vi "Fluence in Tile.vi"(0 "Analyze Fluence in":refnum<class "Analyze Fluence.lvclass">, 5 "Image in":T1, 7 "Energy":dbl, 9 "Create Overlay(T)?":bool, 11 "error in (no error)":errorcluster) -> (4 "Analyze Fluence out":refnum<class "Analyze Fluence.lvclass">, 6 "Image Dst Out":T1, 8 "Max Fluence J/cm^2":dbl, 10 "fluence infos":T2[](array[typedef]), 15 "error out":errorcluster)   [LabVIEW 2014, in "Analyze.lvlib" / "Analyze Fluence.lvclass"]
uses:
  Analyze Fluence.lvclass
  <vilib>/vision/NI_Vision_Development_Module.lvlib
  Fluence Info.ctl
  <vilib>/vision/Image Controls.llb/IMAQ Image.ctl
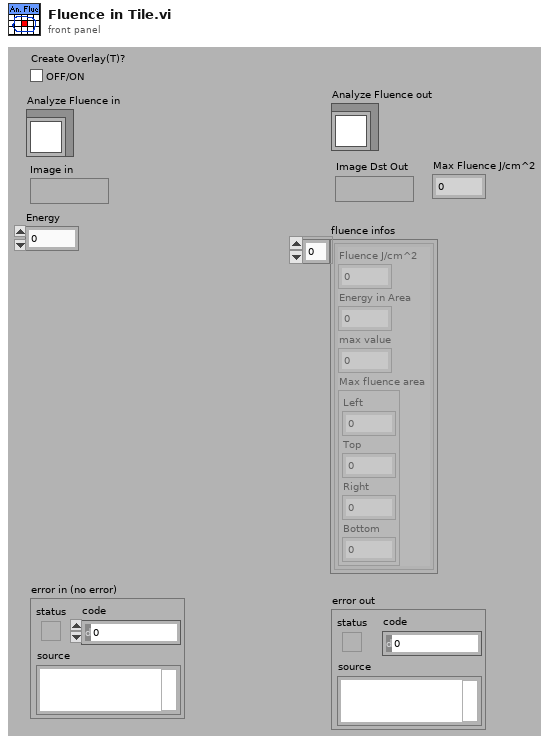
[diagram p1: front panel]
types:
  T1 = typedef "IMAQ Image.ctl" = refnum<image>
  T2 = typedef "Analyze.lvlib/Analyze Fluence.lvclass/Fluence Info.ctl" = cluster{"Fluence J/cm^2":dbl, "Energy in Area":dbl, "max value":i64, "Max fluence area":cluster{"Left":i32, "Top":i32, "Right":i32, "Bottom":i32}}
  T3 = cluster{"Left":i32, "Top":i32, "Right":i32, "Bottom":i32}
  T4 = typedef "Image Type" = u32
  T5 = typedef "ROI Descriptor" = cluster{"Global Rectangle":i32[], "Contours":cluster{"ID":enum32{"External", "Internal"}, "Type":u32, "Coordinates":i32[]}[]}
  T6 = cluster{"Desired Font (Application)":enum16{"User-specified Font", "Application Font", "System Font", "Dialog Font"}, "[User-specified Font]":cluster{"Font Name":string, "Size":i16, "Strikeout?":bool, "Italic?":bool, "Underline?":bool, "Outline?":bool, "Shadow?":bool, "Bold?":bool, "Rotation Angle":dbl}, "Horizontal Alignment":i16, "Vertical Alignment":i16}
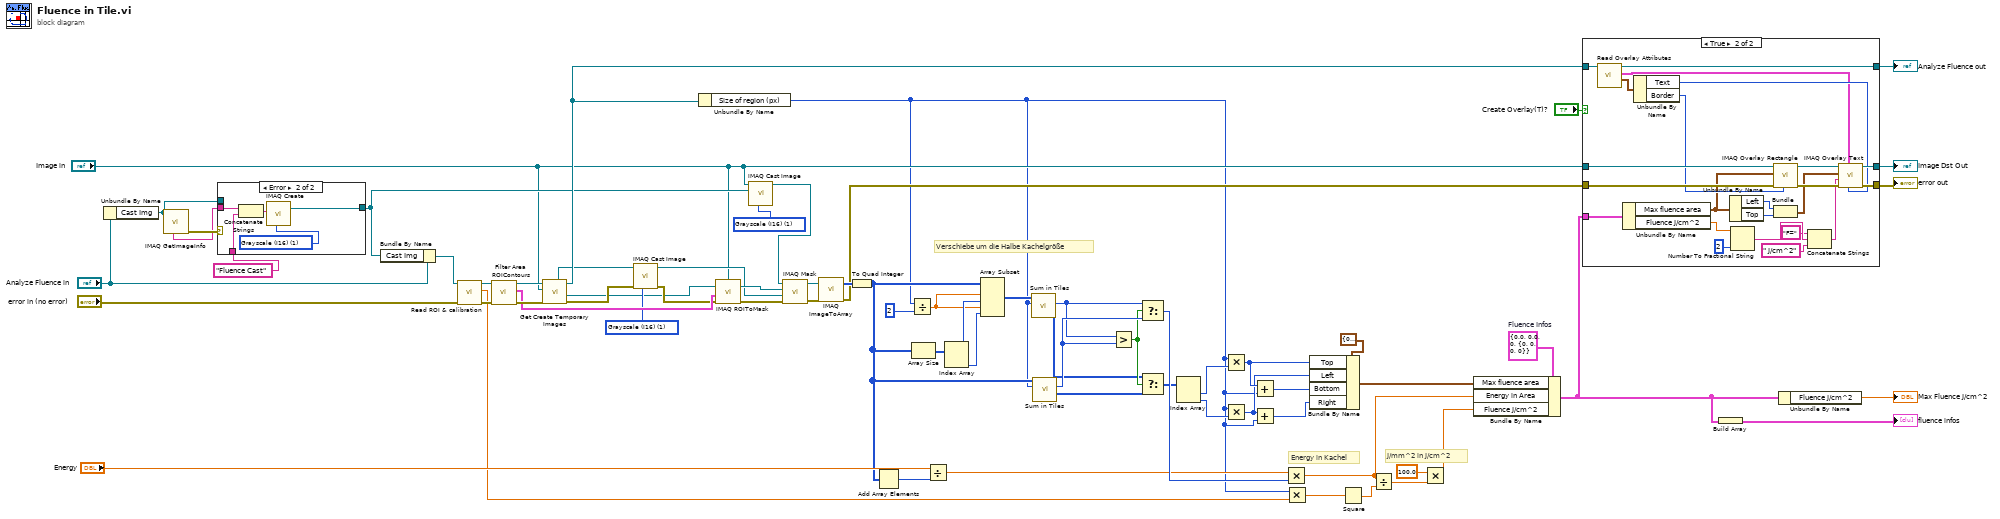
[diagram p0: block diagram]
diagram:
  w8 = T2 {"Fluence J/cm^2"=0.0, "Energy in Area"=0.0, "max value"=0, "Max fluence area"={"Left"=0, "Top"=0, "Right"=0, "Bottom"=0}}  # Fluence Infos
  w44 = T4 1 items=["Grayscale (U8)", "Grayscale (I16)", "Grayscale (SGL)", "Complex (CSG)", "RGB (U32)", "HSL (U32)", "RGB (U64)", "Grayscale (U16)"] ("Image Type")
  w54 = T4 1 items=["Grayscale (U8)", "Grayscale (I16)", "Grayscale (SGL)", "Complex (CSG)", "RGB (U32)", "HSL (U32)", "RGB (U64)", "Grayscale (U16)"] ("Image Type")
  # "Verschiebe um die Halbe Kachelgröße"
  # "J/mm^2 in J/cm^2"
  # "Energy in Kachel"
  n1 = Unbundle By Name("Analyze Fluence in") -> ("Cast Img"=w49:T1)
  n2 = call "IMAQ GetImageInfo"("Image"=w49) -> ("error out"=w52:errorcluster, "Image Name"=w51:string)  [unwired: 3 in, 6 out]
  n3 = case shown="Error" w52 {
    tunnel: w51 -> [_ w77]
    tunnel: "Fluence Cast" -> [_ w75]
    tunnel: [w73 w74] -> w47
    tunnel: w49 -> [w73 _]
    frame No Error {
    }
    frame Error {
      w78 = T4 1 items=["Grayscale (U8)", "Grayscale (I16)", "Grayscale (SGL)", "Complex (CSG)", "RGB (U32)", "HSL (U32)", "RGB (U64)", "Grayscale (U16)"] ("Image Type")
      n4 = Concatenate Strings(w77, w75) -> (w76:string)
      n5 = call "IMAQ Create"("Image Name"=w76, "Image Type"=w78) -> ("New Image"=w74:T1)  [unwired: 3 in, 1 out]
    }
  }
  n6 = Bundle By Name(cluster="Analyze Fluence in", "Cast Img"=w47) -> (w48:refnum<class "Analyze Fluence.lvclass">)
  n7 = call-dynamic "Read ROI & calibration.vi"("error in (no error)"="error in (no error)", "Analyze BaseClass in"=w48) -> ("error out"=w60:errorcluster, "calibration mm/px"=w32:dbl, "Analyze BaseClass out"=w63:refnum<class "Analyze Fluence.lvclass">)  [unwired: 6 in, 1 out]
  n8 = call-dynamic "Filter Area ROIContours.vi"("error in (no error)"=w60, "Analyze BaseClass in"=w63) -> ("error out"=w59:errorcluster, "ROI of Area type"=w56:T5, "Analyze BaseClass out"=w62:refnum<class "Analyze Fluence.lvclass">)  [unwired: 7 in]
  n9 = call-dynamic "Get Create Temporary Images.vi"("error in (no error)"=w59, "Image in"="Image in", "Analyze BaseClass in"=w62) -> ("error out"=w43:errorcluster, "image mask"=w28:T1, "Analyze BaseClass out"=w64:refnum<class "Analyze Fluence.lvclass">, "masked image"=w46:T1)  [unwired: 4 in, 1 out]
  n10 = call "IMAQ Cast Image"("Image Type"=w44, "error in (no error)"=w43, "Image Src"=w46) -> ("error out"=w42:errorcluster, "Image Dst Out"=w45:T1)  [unwired: 7 in]
  n11 = Unbundle By Name(w64) -> ("Size of region (px)"=w9:i32)
  n12 = call "IMAQ ROIToMask"("error in (no error)"=w42, "ROI Descriptor"=w56, "Image"=w28, "Image Model"="Image in") -> ("error out"=w67:errorcluster, "Image Out"=w71:T1)  [unwired: 2 in, 1 out]
  n13 = call "IMAQ Cast Image"("Image Type"=w54, "Image Dst"=w47, "Image Src"="Image in") -> ("Image Dst Out"=w55:T1)  [unwired: 7 in, 1 out]
  n14 = call "IMAQ Mask"("error in (no error)"=w67, "Image Dst"=w45, "Image Mask"=w71, "Image Src"=w55) -> ("error out"=w23:errorcluster, "Image Dst Out"=w24:T1)  [unwired: 1 in]
  n15 = call "IMAQ ImageToArray"("error in (no error)"=w23, "Image"=w24) -> ("error out"=w22:errorcluster, "Image Pixels (I16)"=w58:i16[][])  [unwired: 2 in, 3 out]
  n16 = To Quad Integer(1:w58) -> (0:w57:i64[][])
  n17 = Add Array Elements(numeric array=w57) -> (sum=w41:i64)
  n18 = Divide(x=w9, y=2 ("x")) -> (x/y=w34:dbl)
  n19 = Array Size(array=w57) -> (size(s)=w35:i32[])
  n20 = Divide(x="Energy", y=w41) -> (x/y=w29:dbl)
  n21 = Index Array(array=w35) -> (element #1=w36:i32, element #2=w37:i32)  [unwired: 2 in]
  n22 = Array Subset(array=w57, index (row)=w34, length (row)=w36, index (col)=w34, length (col)=w37) -> (w38:i64[][])
  n23 = call "Sum in Tiles.vi"("size"=w9, "Image"=w38) -> ("Max Index"=w19:i32[], "Maximum"=w39:i64, "Counts in Tiles"=w2:i64[][])  [unwired: 7 in]
  n24 = call "Sum in Tiles.vi"("size"=w9, "Image"=w57) -> ("Max Index"=w18:i32[], "Maximum"=w40:i64, "Counts in Tiles"=w1:i64[][])  [unwired: 7 in]
  n25 = Greater?(x=w39, y=w40) -> (0:w20:bool)
  n26 = Select(t=w39, s=w20, f=w40) -> (s? t:f=w30:i64)
  n27 = Select(t=w19, s=w20, f=w18) -> (s? t:f=w16:i32[])
  n28 = Index Array(array=w16) -> (element #1=w15:i32, element #2=w14:i32)  [unwired: 2 in]
  n29 = Multiply(x=w9, y=w15) -> (x*y=w11:i32)
  n30 = Multiply(x=w9, y=w14) -> (x*y=w10:i32)
  n31 = Add(x=w11, y=w9) -> (x+y=w12:i32)
  n32 = Add(x=w10, y=w9) -> (x+y=w13:i32)
  n33 = Multiply(x=w29, y=w30) -> (x*y=w6:dbl)
  n34 = Multiply(x=w9, y=w32) -> (x*y=w31:dbl)
  n35 = Bundle By Name(cluster=T3 {"Left"=0, "Top"=0, "Right"=0, "Bottom"=0} ("Rectangle"), "Top"=w11, "Left"=w10, "Bottom"=w12, "Right"=w13) -> (w7:T3)
  n36 = Square(x=w31) -> (x^2=w25:dbl)
  n37 = Divide(x=w6, y=w25) -> (x/y=w26:dbl)
  n38 = Multiply(x=100.0, y=w26) -> (x*y=w5:dbl)
  n39 = Bundle By Name(cluster=w8, "Max fluence area"=w7, "Energy in Area"=w6, "Fluence J/cm^2"=w5) -> (w4:T2)
  n40 = case shown="True" "Create Overlay(T)?" {
    tunnel: w4 -> [_ w104]
    tunnel: "Image in" -> [w81 w103]
    tunnel: [w81 w102] -> w69
    tunnel: w22 -> [w80 w101]
    tunnel: [w80 w100] -> w68
    tunnel: [w79 w97] -> w65
    tunnel: w64 -> [w79 w96]
    frame False {
    }
    frame True {
      n41 = call-dynamic "Read Overlay Attributes.vi"("Analyze BaseClass in"=w96) -> ("Overlay colors"=w95:cluster{"Border":u32, "Text":u32}, "Font, Size & Style"=w94:T6, "Analyze BaseClass out"=w97:refnum<class "Analyze Fluence.lvclass">)  [unwired: 7 in, 1 out]
      n42 = Unbundle By Name(w104) -> ("Max fluence area"=w86:T3, "Fluence J/cm^2"=w85:dbl)
      n43 = Unbundle By Name(w95) -> ("Text"=w99:u32, "Border"=w98:u32)
      n44 = Unbundle By Name(w86) -> ("Left"=w87:i32, "Top"=w88:i32)
      n45 = Number To Fractional String(number=w85, precision (6)=i16 2) -> (F-format string=w91:string)  [unwired: 2 in]
      n46 = call "IMAQ Overlay Rectangle"("Color"=w98, "error in (no error)"=w101, "Rectangle"=w86, "Image"=w103) -> ("error out"=w93:errorcluster, "Image Out"=w92:T1)  [unwired: 6 in]
      n47 = Bundle("Left"=w87, "Top"=w88) -> (w89:cluster{"Left":i32, "Top":i32})  [unwired: 1 in]
      n48 = Concatenate Strings("F=" ("string"), w91, " J/cm^2" ("string")) -> (w84:string)
      n49 = call "IMAQ Overlay Text"("Text Color (black)"=w99, "Font, Size & Style"=w94, "error in (no error)"=w93, "String"=w84, "Origin"=w89, "Image"=w92) -> ("error out"=w100:errorcluster, "Image Out"=w102:T1)  [unwired: 4 in]
    }
  }
  "error out" <- w68
  "Image Dst Out" <- w69
  "Analyze Fluence out" <- w65
  n50 = Build Array(w4) -> (→"fluence infos":T2[])
  n51 = Unbundle By Name(w4) -> ("Fluence J/cm^2"=→"Max Fluence J/cm^2":dbl)
